vi "Filename_Sequence_Generator_New.vi"() -> ()   [LabVIEW 2014]
panel:
  out "File Creation Status":errorcluster
  in  "Sampling Time":dbl min=0.0 max=100000.0 step=1.0
  in  "# SnapShots":dbl min=0.0 max=100.0 step=1.0
  out "current time":timestamp
  out "Folder Creation Status":errorcluster
  out "Folder Path":path=path "C:/Users/fzt420/Desktop/Test_Labview/Sample_Mahesh(2)"
  out "New Folder Name Created":string="Sample_Mahesh(2)"
  in  "Give a Sample Name":string
  in  "Choose a Folder to Create":string="Sample_Mahesh(2)"
  in  "Choose the Path":path=path "C:/Users/fzt420/Desktop/Test_Labview"
  # "Procedure to use this VI:\n\n              1) First Choose a File Path where you want to store the Image Snaps taken from the Microscope. \n              \n              2) Now, Choose a Sample_Folder Name for example: \"Sample_Folder\" or any name your are comfortable with.\n\n              3) Then, Choose a Sample_File Name for example: \"Sample_File_Name\" or any name your are comfortable with.\n\n                 ( While Naming the Folders/ Files please use an '_' in place of space. Because it is a good practice of naming files/Folders) \n\n              4) Set how many snapshots you wanna take using the CCD Camera mounted on the Microscope.\n\n              5) Now, set the timer for each SnapShot. Remember: the units of time here is in Milliseconds.    \n\n             6) RUN THE PROGRAM AND SEE THE RESULT in the choosen File Path.\n\nHow this VI Works :\n\n             For example you choose a folder name called \"Sample_Folder\" and File Name Called \"Sample_File_Name\". And, now \n             \n             you choose  no.of snapshots and timer between each snapshot then,  RUN THE VI. \n\n            \n            The Program first tries to see, if there is any folder named \"Sample_Folder\", if there is any folder with the same name\n             in the choosen directory then it creates an another folder incremental version name as \"Sample_Folder(1)\" etc else it\n             creates a folder with a desired name. And after creating an appropriate folder name,  the program then creates a \n             the files as \"Sample_File_Name1\" and so on.\n \n               FOR BETTER UNDERSTANDING PLEASE RUN THE PROGRAM AND SEE THE OUTPUT \n\n            \n             \n\n          \n                                                                                                                                              Mahesh Babu Gorantla\n                                                                                                                                              DURI Intern\n                                                                                                                                              School of Electrical and Computer Engineering \n                                                                                                                                              Purdue University"
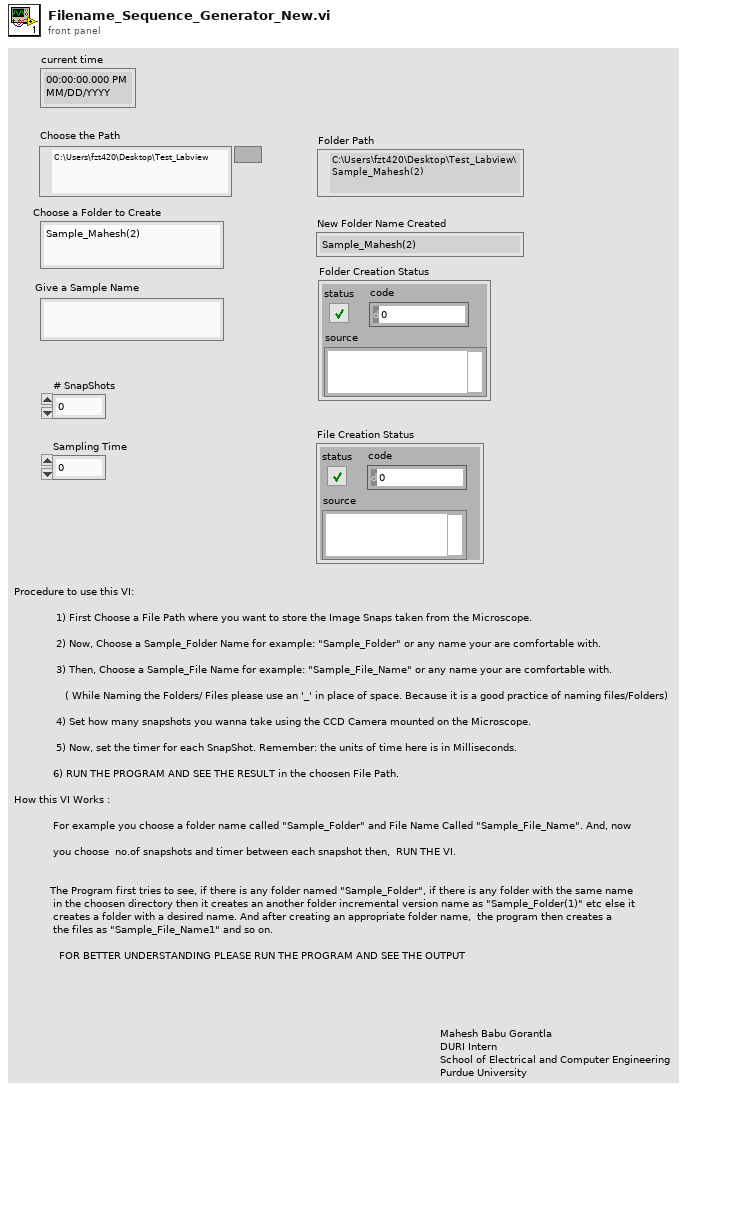
[diagram p1: front panel]
types:
  T1 = enum16{"open", "replace", "create", "open or create", "replace or create", "replace or create with confirmation"}
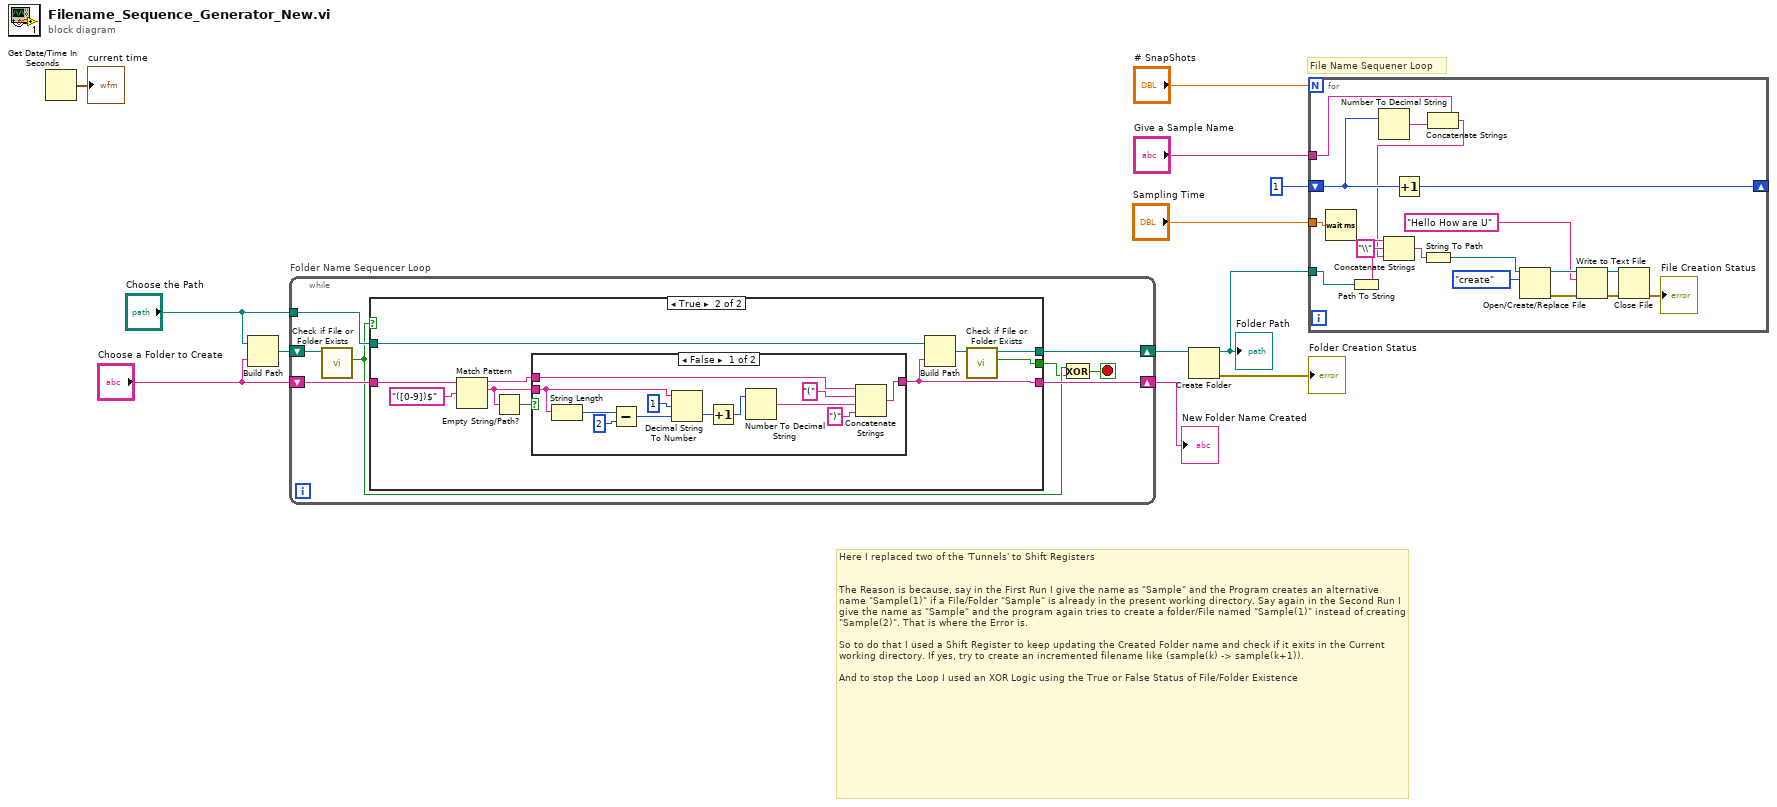
[diagram p0: block diagram]
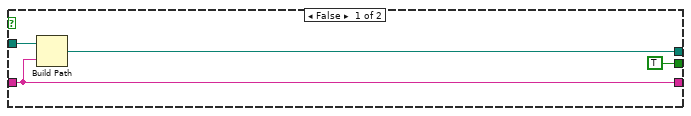
[diagram p2: hidden frame]
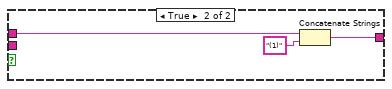
[diagram p3: hidden frame]
diagram:
  # "File Name Sequener Loop"
  # "Here I replaced two of the 'Tunnels' to Shift Registers\n\n\nThe Reason is because, say in the First Run I give the name as \"Sample\" and the Program creates an alternative name \"Sample(1)\" if a File/Folder \"Sample\" is already in the present working directory. Say again in the Second Run I give the name as \"Sample\" and the program again tries to create a folder/File named \"Sample(1)\" instead of creating \"Sample(2)\". That is where the Error is.\n\nSo to do that I used a Shift Register to keep updating the Created Folder name and check if it exits in the Current working directory. If yes, try to create an incremented filename like (sample(k) -> sample(k+1)).  \n\nAnd to stop the Loop I used an XOR Logic using the True or False Status of File/Folder Existence"
  n1 = Get Date/Time In Seconds() -> (seconds since 1Jan1904=→"current time":timestamp)
  n2 = Build Path(base path="Choose the Path", name or relative path="Choose a Folder to Create") -> (appended path=w9:path)
  n3 = while "Folder Name Sequencer Loop" {
    tunnel: "Choose the Path" -> [w17]
    shift-right: [w19] -> w8
    shift-left: w9 -> [w16]
    shift-right: [w20] -> w12
    shift-left: "Choose a Folder to Create" -> [w18]
    stop <- w13 stop-if-true
    n4 = call <vilib>:"Check if File or Folder Exists.vi"("path"=w16) -> ("file or folder exists?"=w15:bool)  [unwired: 8 in, 2 out]
    n5 = case shown="True" w15 {
      tunnel: w18 -> [w23 w34]
      tunnel: [w23 w25] -> w20
      tunnel: [w22 w27] -> w19
      tunnel: w17 -> [w24 w29]
      tunnel: [TRUE w26] -> w14
      frame False {
        n6 = Build Path(base path=w24, name or relative path=w23) -> (appended path=w22:path)
      }
      frame True {
        n7 = Match Pattern(string=w34, regular expression="([0-9])$") -> (before substring=w31:string, match substring=w30:string)  [unwired: 1 in, 2 out]
        n8 = Empty String/Path?(string/path=w30) -> (empty?=w32:bool)
        n9 = case shown="False" w32 {
          tunnel: w31 -> [w39 w49]
          tunnel: w30 -> [w42 _]
          tunnel: [w35 w47] -> w25
          frame False {
            n10 = String Length(string=w42) -> (length=w46:i32)
            n11 = Subtract(x=w46, y=2) -> (x-y=w44:i32)
            n12 = Decimal String To Number(string=w42, offset=1, default (0L)=w44) -> (number=w41:i32)  [unwired: 1 out]
            n13 = Increment(x=w41) -> (x+1=w40:i32)
            n14 = Number To Decimal String(number=w40) -> (decimal integer string=w38:string)  [unwired: 1 in]
            n15 = Concatenate Strings(w39, "(" ("string"), w38, ")" ("string")) -> (w35:string)
          }
          frame True {
            n16 = Concatenate Strings(w49, "(1)" ("string")) -> (w47:string)
          }
        }
        n17 = Build Path(base path=w29, name or relative path=w25) -> (appended path=w28:path)
        n18 = call <vilib>:"Check if File or Folder Exists.vi"("path"=w28) -> ("file or folder exists?"=w26:bool, "dup path"=w27:path)  [unwired: 8 in, 1 out]
      }
    }
    n19 = Exclusive Or(1:w14, 2:w15) -> (0:w13:bool)
  }
  "New Folder Name Created" <- w12
  n20 = Create Folder(path (use dialog)=w8) -> (created path=w1:path, error out=→"Folder Creation Status":errorcluster)  [unwired: 2 in, 1 out]
  "Folder Path" <- w1
  n21 = for {
    N: "# SnapShots" -> [_]
    tunnel: "Sampling Time" -> [w67]
    tunnel: "Give a Sample Name" -> [w59]
    shift-right: [w66] -> _
    shift-left: 1 -> [w60]
    tunnel: w1 -> [w54]
    n22 = Wait (ms)(milliseconds to wait=w67) -> ()  [unwired: 1 out]
    n23 = Path To String(path=w54) -> (string=w55:string)
    n24 = Number To Decimal String(number=w60) -> (decimal integer string=w58:string)  [unwired: 1 in]
    n25 = Increment(x=w60) -> (x+1=w66:i32)
    n26 = Concatenate Strings(w59, w58) -> (w51:string)
    n27 = Concatenate Strings(w55, "\\" ("string"), w51) -> (w57:string)
    n28 = String To Path(string=w57) -> (path=w56:path)
    n29 = Open/Create/Replace File(file path (use dialog)=w56, operation (0:open)=T1."create") -> (refnum out=w65:refnum<file>, error out=w63:errorcluster)  [unwired: 4 in, 1 out]
    n30 = Write to Text File(file (use dialog)=w65, text="Hello How are U", error in=w63) -> (refnum out=w64:refnum<file>, error out=w62:errorcluster)  [unwired: 1 in, 1 out]
    n31 = Close File(refnum=w64, error in=w62) -> (error out=→"File Creation Status":errorcluster)  [unwired: 1 out]
  }
